vi "script_get_next_line.vi"(2 "Value 2":i32, 3 "Value 3":string[](array[string])) -> (0 "String":string, 1 "Value":i32)   [LabVIEW 2010]
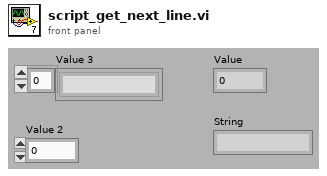
[diagram p1: front panel]
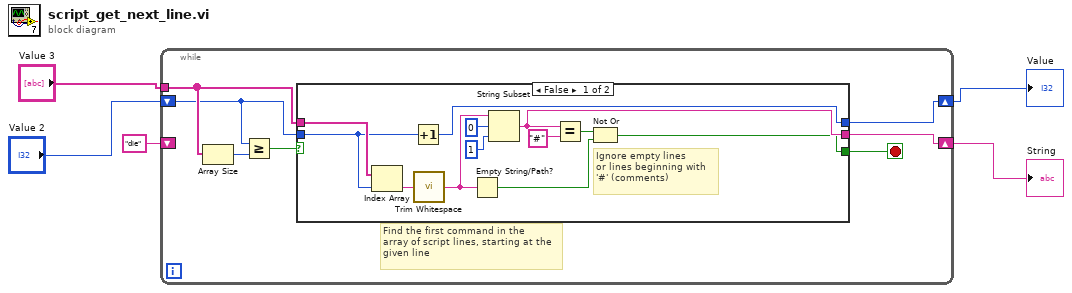
[diagram p0: block diagram]
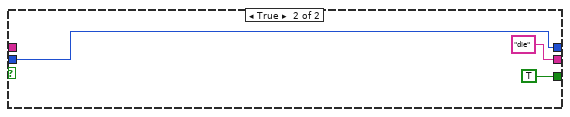
[diagram p2: hidden frame]
diagram:
  n1 = while {
    tunnel: "Value 3" -> [w9]
    shift-right: [w8] -> w3
    shift-left: "die" -> [_]
    shift-right: [w6] -> w5
    shift-left: "Value 2" -> [w7]
    stop <- w10 stop-if-true
    # "Find the first command in the\narray of script lines, starting at the\ngiven line"
    n2 = Array Size(array=w9) -> (size(s)=w12:i32)
    n3 = Greater Or Equal?(x=w7, y=w12) -> (x >= y?=w11:bool)
    n4 = case shown="False" w11 {
      tunnel: [w16 "die"] -> w8
      tunnel: [w13 TRUE] -> w10
      tunnel: w9 -> [w24 _]
      tunnel: w7 -> [w15 w25]
      tunnel: [w14 w25] -> w6
      frame False {
        # "Ignore empty lines\nor lines beginning with\n'#' (comments)"
        n5 = Index Array(array=w24, index=w15) -> (element=w23:string)
        n6 = Increment(x=w15) -> (x+1=w14:i32)
        n7 = call <vilib>:"Trim Whitespace.vi"("string"=w23) -> ("trimmed string"=w18:string)  [unwired: 1 in]
        n8 = Empty String/Path?(string/path=w18) -> (empty?=w17:bool)
        n9 = String Subset(string=w18, offset (0)=0, length (rest)=1 ("length (rest)")) -> (substring=w16:string)
        n10 = Equal?(x=w16, y="#") -> (x = y?=w19:bool)
        n11 = Not Or(1:w17, 2:w19) -> (0:w13:bool)
      }
      frame True {
      }
    }
  }
  "Value" <- w5
  "String" <- w3
